vi "Read Multi-Channel Waveform.vi"(8 "error in (no error)":errorcluster, 10 "Channels":T1[](array[typedef]), 11 "PicoScope 3000a in":refnum<class "PicoScope 3000a.lvclass">) -> (0 "error out":errorcluster, 2 "Waveform":waveform(dbl)[](graph), 3 "PicoScope 3000a out":refnum<class "PicoScope 3000a.lvclass">)   [LabVIEW 2018, in "PicoScope 3000a.lvlib" / "PicoScope 3000a.lvclass"]
doc: "This Override method is used to initiate multi-channel waveform acquisition. Select targeted channels at the 'Channels' control and output waveform data to the 'Waveform' indicator."
uses:
  PicoScope 3000a.lvclass
  PPLs/Oscilloscope/Parent/Oscilloscope.lvlibp/Custom Controls/Analog Channels.ctl
  PicoScope 3000a.lvclass/PicoScope 3000a.ctl
  <instrlib>/PicoScope/PicoScope.lvlib
  PPLs/Oscilloscope/Parent/Oscilloscope.lvlibp
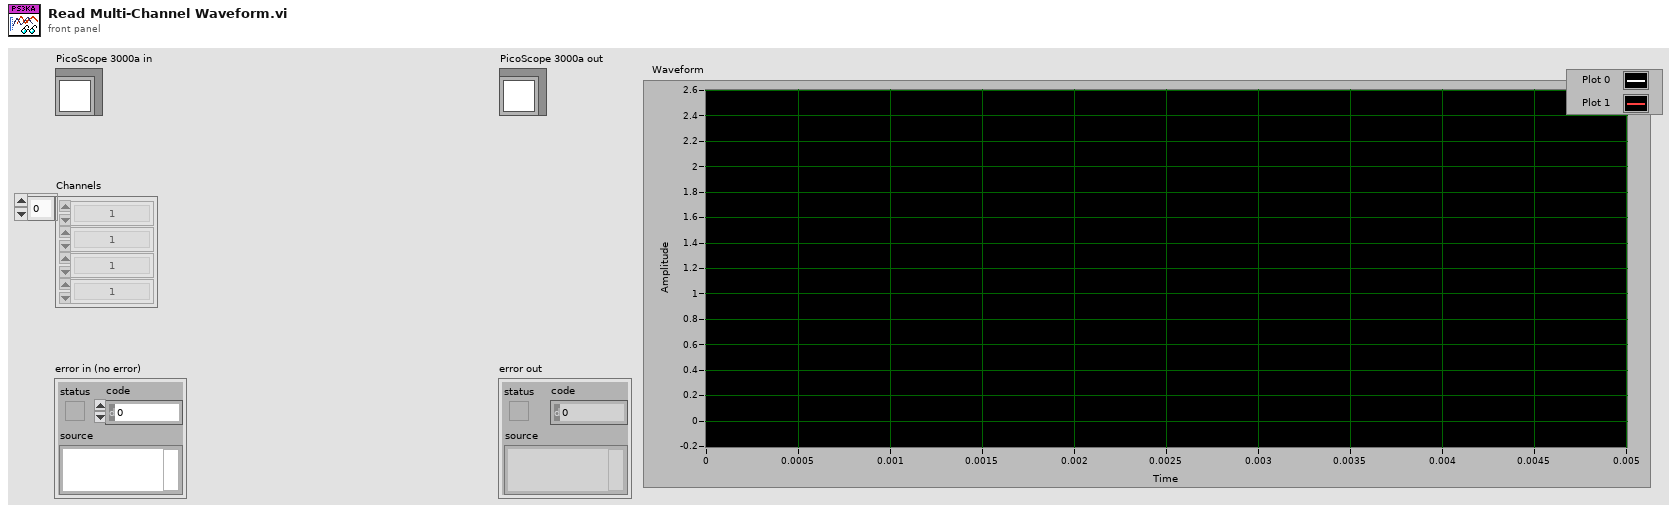
[diagram p1: front panel]
types:
  T1 = typedef "Oscilloscope.lvlibp/Analog Channels.ctl" = enum16{"1", "2", "3", "4", "5", "6", "7", "8", "9", "10", "11", "12", "13", "14", "15", "16"}
  T2 = cluster{"preTriggerSamples":u32, "postTriggerSamples":u32, "timebase":u32, "Down-Sample Mode":i32, "Down Sample Ratio":u32, "Four Channel Device":bool}
  T3 = cluster{"Driver Version":string, "USB Version":string, "Hardware":string, "Variant":string, "Batch and Serial":string, "Cal Date":string, "Kernel Version":string, "Digital HW Version":string, "Analogue HW Version":string, "MSO":bool, "Number of channels":i16}
  T4 = cluster{"preTriggerSamples":u32, "postTriggerSamples":u32, "timebase":u32, "Down-Sample Mode":i32, "Down Sample Ratio":u32}
  T5 = cluster{"Channel":enum16{"CH. A", "CH. B", "CH. C", "CH. D"}, "Range":u32}[]
  T6 = cluster{"Enabled":bool, "Coupling":u32, "Range":u32, "Analogue Offset":sgl}[]
  T7 = cluster{"Sample Frequency":sgl, "Sample Rate":sgl, "Max Samples Available":i32, "Number of Samples":u32, "Total Capture Time (sec) ":sgl, "Max Total Capture Time Available (sec)":sgl}
  T8 = cluster{"Enabled":bool, "Coupling":u32, "Range":u32, "Analogue Offset":sgl}
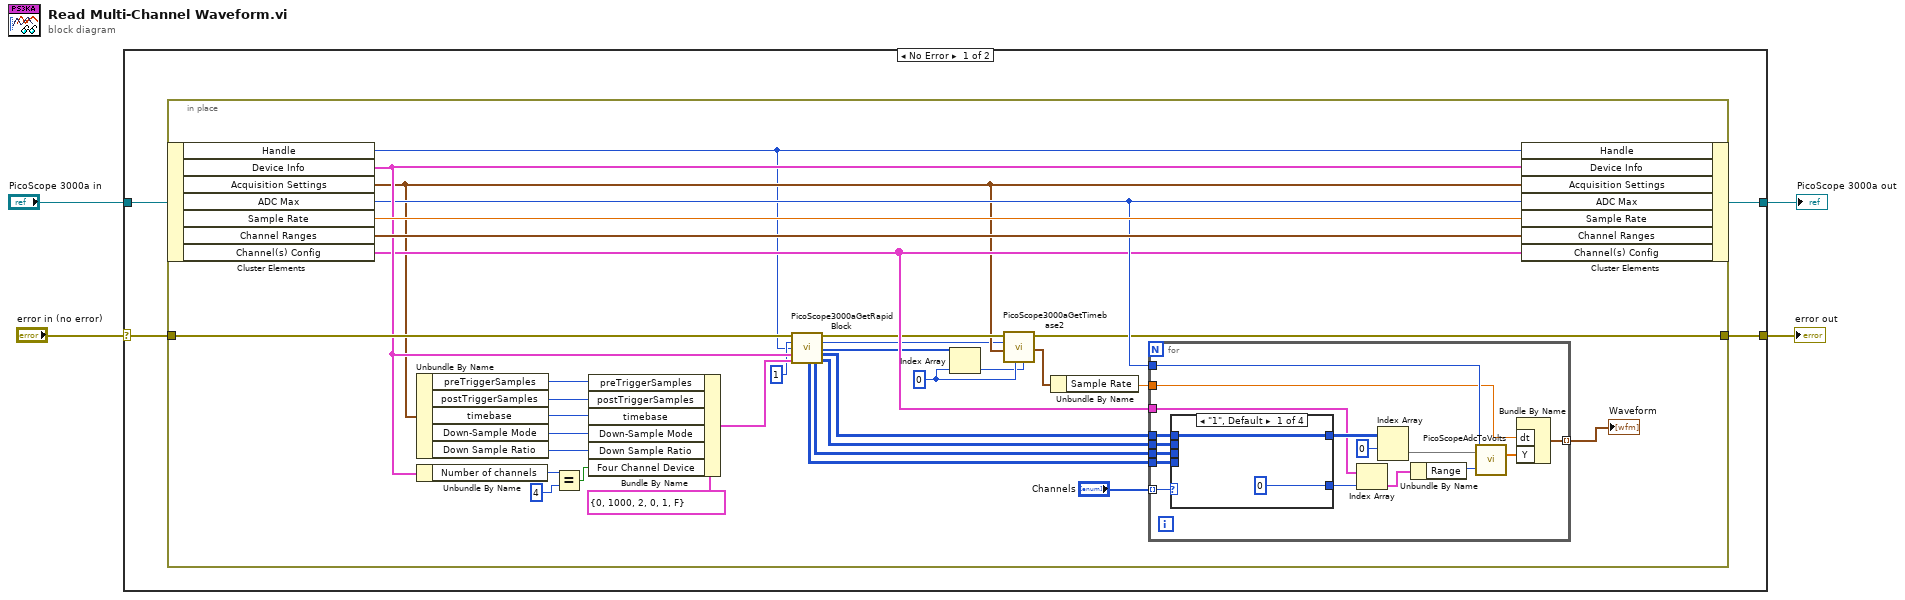
[diagram p0: block diagram]
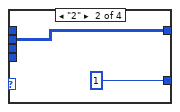
[diagram p2: hidden frame]
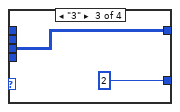
[diagram p3: hidden frame]
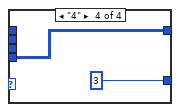
[diagram p4: hidden frame]
diagram:
  n1 = case shown="No Error" "error in (no error)" {
    selector: "error in (no error)" -> [w7 w66]
    tunnel: "PicoScope 3000a in" -> [w8 w67]
    tunnel: [w5 w66] -> w1
    tunnel: [w6 w67] -> w3
    frame No Error {
      n2 = in-place {
        in-place-border: w7 -> [w39]
        in-place-border: [w16] -> w5
        w12 = 0 ("index")
        n3 = in-place-cluster #1(w8) -> ("Handle"=w10:i16, "Device Info"=w32:T3, "Acquisition Settings"=w14:T4, "ADC Max"=w20:i16, "Sample Rate"=w41:sgl, "Channel Ranges"=w40:T5, "Channel(s) Config"=w19:T6)
        n4 = Unbundle By Name(w14) -> ("preTriggerSamples"=w37:u32, "postTriggerSamples"=w36:u32, "timebase"=w35:u32, "Down-Sample Mode"=w34:i32, "Down Sample Ratio"=w33:u32)
        n5 = Unbundle By Name(w32) -> ("Number of channels"=w31:i16)
        n6 = Equal?(x=w31, y=i16 4) -> (x = y?=w29:bool)
        n7 = Bundle By Name(cluster=T2 {"preTriggerSamples"=0, "postTriggerSamples"=1000, "timebase"=2, "Down-Sample Mode"=0, "Down Sample Ratio"=1, "Four Channel Device"=FALSE} ("Rapid Block Acquisition Settings"), "preTriggerSamples"=w37, "postTriggerSamples"=w36, "timebase"=w35, "Down-Sample Mode"=w34, "Down Sample Ratio"=w33, "Four Channel Device"=w29) -> (w28:T2)
        n8 = call <instrlib>:"PicoScope3000aGetRapidBlock.vi"("error in"=w39, "Number of Segments"=u32 1, "handle in"=w10, "Device Info"=w32, "Rapid Block Acquisition Settings"=w28) -> ("Channel A Buffer"=w25:i16[][], "Channel B Buffer"=w24:i16[][], "error out"=w17:errorcluster, "handle out"=w9:i16, "noOfSamples Array"=w13:u32[], "Channel C Buffer"=w23:i16[][], "Channel D Buffer"=w22:i16[][])  [unwired: 2 in, 2 out]
        n9 = Index Array(array=w13, index=w12) -> (element=w11:u32)
        n10 = call <instrlib>:"PicoScope3000aGetTimebase2.vi"("Number of Samples"=w11, "Memory Segment"=w12, "Acquisition Settings"=w14, "handle in"=w9, "error in (no error)"=w17) -> ("error out"=w16:errorcluster, "Properties Panel"=w21:T7)  [unwired: 4 in, 1 out]
        n11 = Unbundle By Name(w21) -> ("Sample Rate"=w15:sgl)
        n12 = for {
          tunnel: "Channels" -> [w57] mode=indexing
          tunnel: w25 -> [w56]
          tunnel: w24 -> [w52]
          tunnel: w23 -> [w51]
          tunnel: w22 -> [w50]
          tunnel: w15 -> [w43]
          tunnel: w20 -> [w49]
          tunnel: w19 -> [w45]
          tunnel: [w42] -> w18 mode=indexing
          n13 = case shown="\"1\", Default" w57 {
            tunnel: w56 -> [w59 _ _ _]
            tunnel: [w59 w61 w63 w65] -> w54
            tunnel: w52 -> [_ w61 _ _]
            tunnel: w51 -> [_ _ w63 _]
            tunnel: w50 -> [_ _ _ w65]
            tunnel: [0 1 2 3] -> w48
            frame "1", Default {
            }
            frame "2" {
            }
            frame "3" {
            }
            frame "4" {
            }
          }
          n14 = Index Array(array=w45, index=w48) -> (element=w47:T8)
          n15 = Index Array(array=w54, index (row)=0) -> (element=w53:i16[])  [unwired: 1 in]
          n16 = Unbundle By Name(w47) -> ("Range"=w46:u32)
          n17 = call <instrlib>:"PicoScopeAdcToVolts.vi"("Max_adc"=w49, "Range Index"=w46, "Data"=w53) -> ("Data (Volts)"=w44:dbl[])
          n18 = Bundle By Name("dt"=w43, "Y"=w44) -> (w42:waveform(dbl))  [unwired: 1 in]
        }
        "Waveform" <- w18
        n19 = in-place-cluster #1("Handle"=w10, "Device Info"=w32, "Acquisition Settings"=w14, "ADC Max"=w20, "Sample Rate"=w41, "Channel Ranges"=w40, "Channel(s) Config"=w19) -> (w6:refnum<class "PicoScope 3000a.lvclass">)
      }
    }
    frame Error {
    }
  }
  "error out" <- w1
  "PicoScope 3000a out" <- w3
